vi "TransferItems.vi"(8 "error in (no error)":errorcluster, 10 "Session":refnum<class "Session.lvclass">, 11 "TranferFiles-Put in":refnum<class "TranferFiles-Put.lvclass">) -> (0 "error out":errorcluster, 3 "TranferFiles-Put out":refnum<class "TranferFiles-Put.lvclass">)   [LabVIEW 2015, in "WinSCP.lvlib" / "TranferFiles-Put.lvclass"]
uses:
  TranferFiles-Put.lvclass
  Session/Session.lvclass
  C:/Program Files (x86)/WinSCP/WinSCPnet.dll
  Program Files (x86)/WinSCP/WinSCPnet.dll
  FileTransferOptions/FileTransferOptions.lvclass
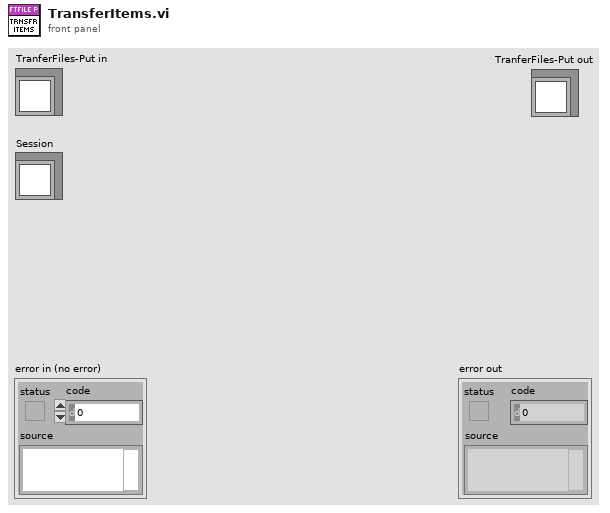
[diagram p1: front panel]
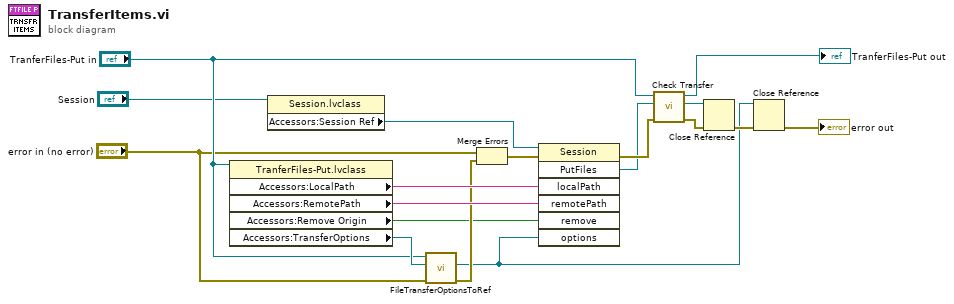
[diagram p0: block diagram]
diagram:
  n1 = property class="TranferFiles-Put.lvclass"(reference="TranferFiles-Put in") -> ("Accessors:LocalPath"=w17:string, "Accessors:RemotePath"=w16:string, "Accessors:Remove Origin"=w3:bool, "Accessors:TransferOptions"=w12:refnum<class "FileTransferOptions.lvclass">)  [unwired: 1 in, 2 out]
  n2 = property class="Session.lvclass"(reference="Session") -> ("Accessors:Session Ref"=w14:refnum<k24>)  [unwired: 1 in, 2 out]
  n3 = call-dynamic "FileTransferOptionsToRef.vi"("error in (no error)"="error in (no error)", "FileTransferOptions"=w12, "FileTransfer in"="TranferFiles-Put in") -> ("error out"=w10:errorcluster, "TransferOptions Ref"=w2:refnum<k24>)  [unwired: 7 in]
  n4 = Merge Errors("error in (no error)", w10) -> (w11:errorcluster)
  n5 = invoke class="Session" method="PutFiles"(reference=w14, error in=w11, "localPath"=w17, "remotePath"=w16, "remove"=w3, "options"=w2) -> (error out=w18:errorcluster, "PutFiles"=w1:refnum<k24>)  [unwired: 1 in, 5 out]
  n6 = call-dynamic "Check Transfer.vi"("error in"=w18, "TransferOperationResult in"=w1, "FileTransfer in"="TranferFiles-Put in") -> ("error out"=w15:errorcluster, "TransferOperationResult out"=w13:refnum<k24>, "FileTransfer out"=→"TranferFiles-Put out":refnum<class "TranferFiles-Put.lvclass">)  [unwired: 6 in]
  n7 = Close Reference(reference=w13, error in (no error)=w15) -> (error out=w9:errorcluster)
  n8 = Close Reference(reference=w2, error in (no error)=w9) -> (error out=→"error out":errorcluster)
